vi "decodeStream.vi"(8 "error in (no error)":errorcluster, 9 "beginIndex":i32, 10 "binary stream in":u8[](array[numeric]) format="%.0x", 11 "tBSONString in":refnum<class "tBSONString.lvclass">) -> (0 "error out":errorcluster, 1 "endIndex":i32, 2 "binary stream out":u8[](array[numeric]), 3 "tBSONString out":refnum<class "tBSONString.lvclass">)   [LabVIEW 2013, in "BSON.lvlib" / "tBSONString.lvclass"]
uses:
  tBSONString.lvclass
  tBSONElement/tBSONElement.lvclass
  setValue.vi
  BSON.lvlib
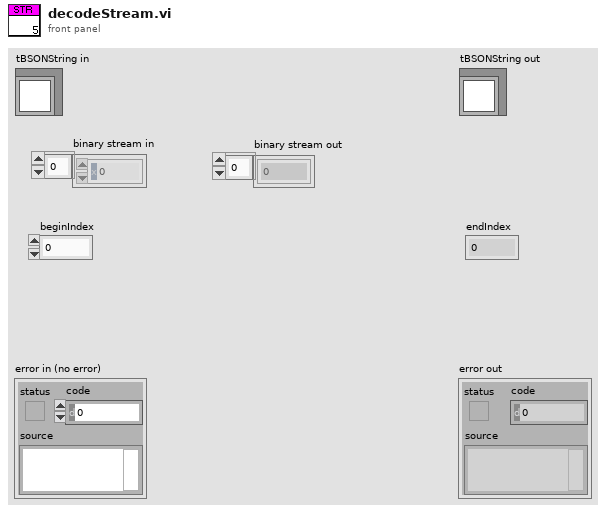
[diagram p1: front panel]
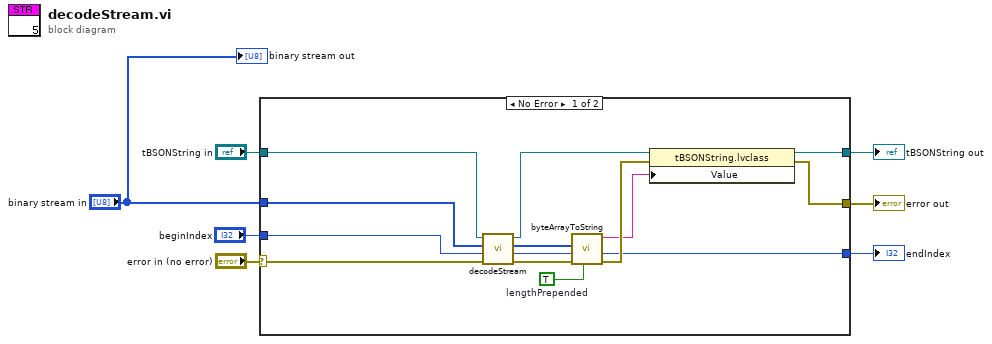
[diagram p0: block diagram]
diagram:
  n1 = case shown="No Error" "error in (no error)" {
    selector: "error in (no error)" -> [w21 w24]
    tunnel: [w20 w24] -> w6
    tunnel: "tBSONString in" -> [w19 w23]
    tunnel: [w17 w23] -> w4
    tunnel: "binary stream in" -> [w18 _]
    tunnel: "beginIndex" -> [w16 w22]
    tunnel: [w8 w22] -> w1
    frame No Error {
      w12 = TRUE  # lengthPrepended
      n2 = call-parent "decodeStream.vi"("error in (no error)"=w21, "beginIndex"=w16, "binary stream"=w18, "tBSONElement in"=w19) -> ("error out"=w14:errorcluster, "endIndex"=w11:i32, "binary stream out"=w10:u8[], "tBSONElement out"=w15:refnum<class "tBSONString.lvclass">)  [unwired: 4 in]
      n3 = call "byteArrayToString.vi"("lengthPrepended"=w12, "error in (no error)"=w14, "startIndex"=w11, "ByteArrayIn"=w10) -> ("error out"=w13:errorcluster, "endIndex"=w8:i32, "String"=w9:string)  [unwired: 4 in, 1 out]
      n4 = property class="tBSONString.lvclass"(reference=w15, error in=w13, "Value"=w9) -> (reference out=w17:refnum<class "tBSONString.lvclass">, error out=w20:errorcluster)
    }
    frame Error {
    }
  }
  "error out" <- w6
  "tBSONString out" <- w4
  "endIndex" <- w1
  "binary stream out" <- "binary stream in"
